vi "CreateInterface.vi"(8 "error in (no error)":errorcluster, 9 "InterfaceInfo":T1) -> (0 "error out":errorcluster, 1 "handle":i64 format="%x", 2 "function return":u32)   [LabVIEW 2013, in "MvCameraControl.lvlib"]
doc: "MV_CAMCTRL_API int __stdcall MV_CC_CreateInterface(IN OUT void ** handle, IN MV_INTERFACE_INFO* pInterfaceInfo);"
uses:
  MvCameraControl.lvlib
  MvCameraPatch.dll
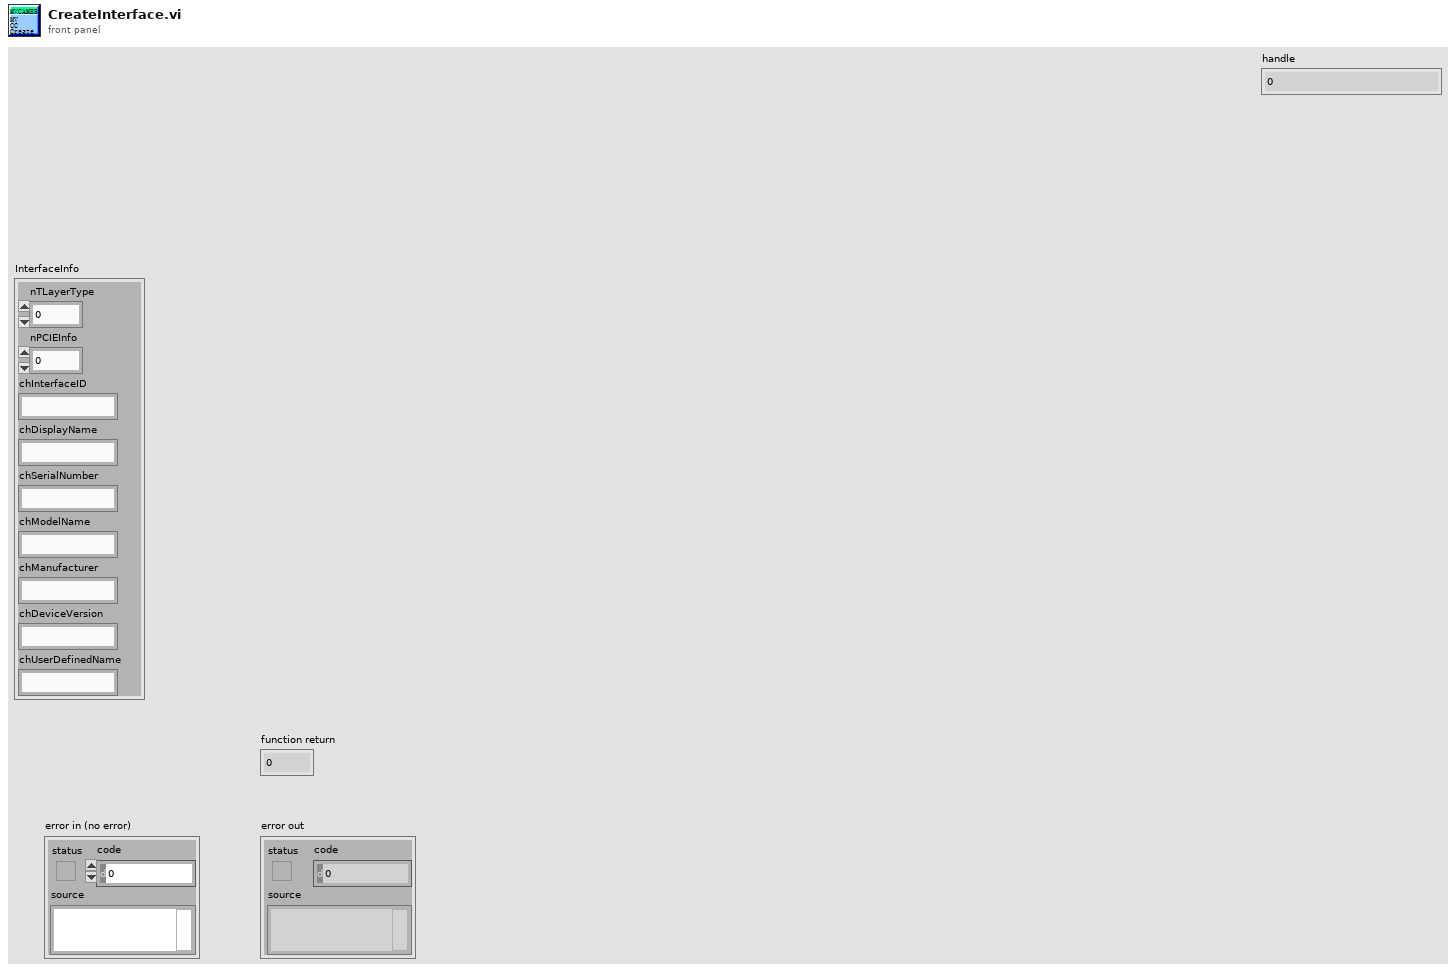
[diagram p1: front panel]
types:
  T1 = cluster{"nTLayerType":u32, "nPCIEInfo":u32, "chInterfaceID":string, "chDisplayName":string, "chSerialNumber":string, "chModelName":string, "chManufacturer":string, "chDeviceVersion":string, "chUserDefinedName":string}
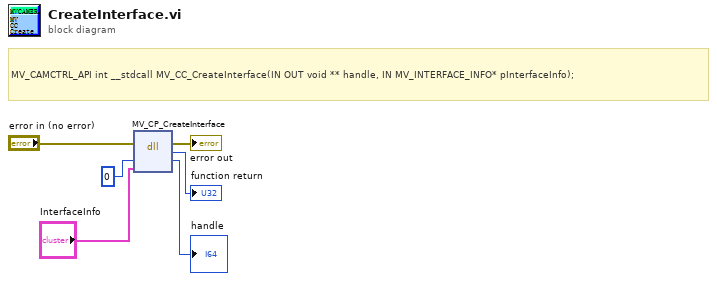
[diagram p0: block diagram]
diagram:
  # "MV_CAMCTRL_API int __stdcall MV_CC_CreateInterface(IN OUT void ** handle, IN MV_INTERFACE_INFO* pInterfaceInfo);"
  n1 = dll-call lib="MvCameraPatch.dll" fn="MV_CP_CreateInterface"(error in="error in (no error)", "handle"=0, "pInterfaceInfo"="InterfaceInfo") -> (error out=→"error out":errorcluster, "return type"=→"function return":i32, "handle"=→"handle":i64)  [unwired: 3 in, 1 out]
